vi "Write Grid Summary.vi"(8 "error in (no error)":errorcluster, 10 "Grid Summary":T1, 11 "Module Data in":refnum<class "Grassfire Algorithm.lvclass">) -> (0 "error out":errorcluster, 3 "Module Data out":refnum<class "Grassfire Algorithm.lvclass">)   [LabVIEW 2019, in "Grassfire Algorithm.lvclass"]
uses:
  Grassfire Algorithm.lvclass
  Grid Summary--cluster.ctl
  Index Column Row--cluster.ctl
  Grassfire Algorithm.lvclass/Grassfire Algorithm.ctl
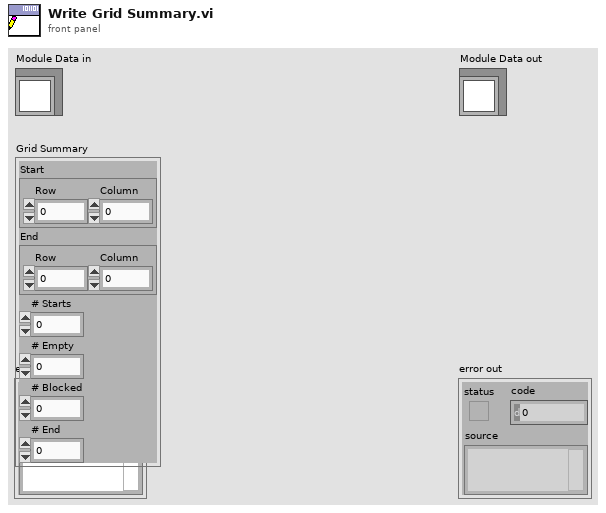
[diagram p1: front panel]
types:
  T1 = typedef "Grassfire Algorithm.lvclass/Grid Summary--cluster.ctl" = cluster{"Start":T2, "End":T2, "# Starts":i32, "# Empty":i32, "# Blocked":i32, "# End":i32}
  T2 = typedef "Grassfire Algorithm.lvclass/Index Column Row--cluster.ctl" = cluster{"Row":i32, "Column":i32}
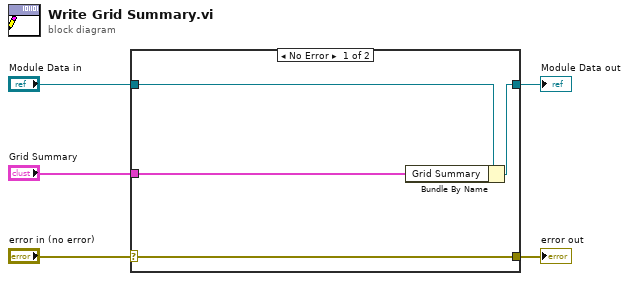
[diagram p0: block diagram]
diagram:
  n1 = case shown="No Error" "error in (no error)" {
    selector: "error in (no error)" -> [w9 w10]
    tunnel: [w9 w10] -> w4
    tunnel: [w7 w11] -> w2
    tunnel: "Module Data in" -> [w8 w11]
    tunnel: "Grid Summary" -> [w6 _]
    frame No Error {
      n2 = Bundle By Name(cluster=w8, "Grid Summary"=w6) -> (w7:refnum<class "Grassfire Algorithm.lvclass">)
    }
    frame Error {
    }
  }
  "error out" <- w4
  "Module Data out" <- w2
